vi "Before Each.vi"(8 "Error In":errorcluster) -> (0 "Error Out":errorcluster, 3 "Writer Out":refnum<class "Writer.lvclass">)   [LabVIEW 2018, in "Tests.lvlib" / "Writer.lvlib"]
uses:
  Writer.lvlib
  src/LabPack/Public/Writer/Writer.lvclass
  src/LabPack/Public/Writer/Private/Begin by Value.vi
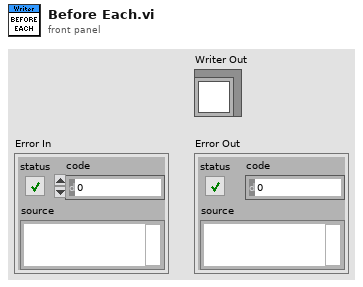
[diagram p1: front panel]
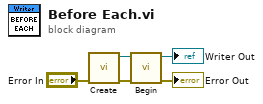
[diagram p0: block diagram]
diagram:
  n1 = call "Create.vi"("Error In"="Error In") -> ("Error Out"=w5:errorcluster, "Writer"=w3:refnum<class "Writer.lvclass">)  [unwired: 9 in]
  n2 = call-poly "Begin.vi"("Error In"=w5, "Writer In"=w3) -> ("Error Out"=→"Error Out":errorcluster, "Writer Out"=→"Writer Out":refnum<class "Writer.lvclass">)  [unwired: 8 in]
